vi "include mapping.vi"(9 "is mapped?":bool, 10 "get unmapped?":bool, 11 "get mapped?":bool) -> (2 "include?":bool)   [LabVIEW 2016, in "FPGA Resource Manager System Definition.lvlib"]
uses:
  FPGA Resource Manager System Definition.lvlib
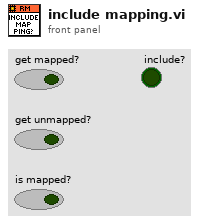
[diagram p1: front panel]
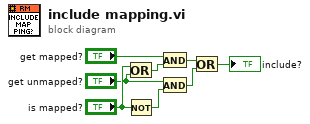
[diagram p0: block diagram]
diagram:
  n1 = Or(x="is mapped?", y="get unmapped?") -> (x .or. y?=w8:bool)
  n2 = Not(x="is mapped?") -> (.not. x?=w5:bool)
  n3 = And(x="get mapped?", y=w8) -> (x .and. y?=w3:bool)
  n4 = And(x="get unmapped?", y=w5) -> (x .and. y?=w2:bool)
  n5 = Or(x=w3, y=w2) -> (x .or. y?=→"include?":bool)
